vi "Teleop Points.vi"(0 "Char in":i16, 7 "Error In":errorcluster) -> (11 "Error Out":errorcluster, 17 "Bottom Goal":dbl, 18 "Top Goal":dbl, 19 "Assists":dbl)   [LabVIEW 2013]
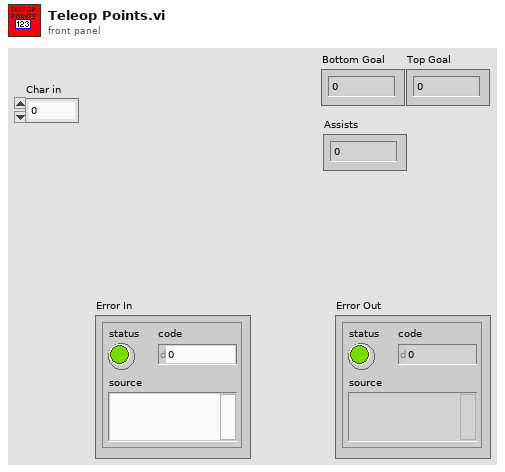
[diagram p1: front panel]
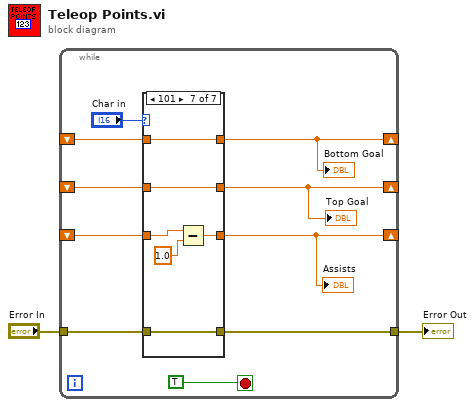
[diagram p0: block diagram]
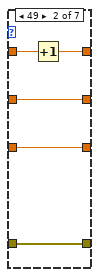
[diagram p3: hidden frame]
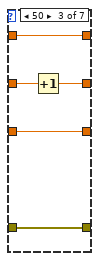
[diagram p4: hidden frame]
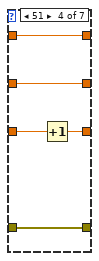
[diagram p5: hidden frame]
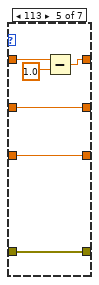
[diagram p6: hidden frame]
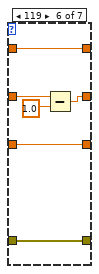
[diagram p7: hidden frame]
diagram:
  n1 = while {
    shift-right: [w5] -> _
    shift-left: _ -> [w10]
    shift-right: [w6] -> _
    shift-left: _ -> [w9]
    tunnel: "Error In" -> [w8]
    tunnel: [w7] -> w1
    shift-right: [w3] -> _
    shift-left: _ -> [w4]
    stop <- TRUE stop-if-true
    n2 = case shown="101" "Char in" {
      tunnel: w10 -> [w16 w21 w26 w31 w36 w43 w49]
      tunnel: w9 -> [w15 w19 w25 w30 w34 w41 w48]
      tunnel: [w16 w20 w26 w31 w35 w43 w49] -> w5
      tunnel: [w15 w19 w24 w30 w34 w40 w48] -> w6
      tunnel: w8 -> [w14 w18 w23 w27 w33 w39 w44]
      tunnel: [w14 w18 w23 w27 w33 w39 w44] -> w7
      tunnel: w4 -> [w13 w17 w22 w29 w32 w38 w46]
      tunnel: [w13 w17 w22 w28 w32 w38 w45] -> w3
      frame 0, Default {
      }
      frame 49 {
        n3 = Increment(x=w21) -> (x+1=w20:dbl)
      }
      frame 50 {
        n4 = Increment(x=w25) -> (x+1=w24:dbl)
      }
      frame 51 {
        n5 = Increment(x=w29) -> (x+1=w28:dbl)
      }
      frame 113 {
        n6 = Subtract(x=w36, y=1.0) -> (x-y=w35:dbl)
      }
      frame 119 {
        n7 = Subtract(x=w41, y=1.0) -> (x-y=w40:dbl)
      }
      frame 101 {
        n8 = Subtract(x=w46, y=1.0) -> (x-y=w45:dbl)
      }
    }
    "Top Goal" <- w6
    "Bottom Goal" <- w5
    "Assists" <- w3
  }
  "Error Out" <- w1
